vi "changeTempdatabase.vi"(3 "Database input(hidden)":T1={"DB name"="K2_r01", "UID"="mgupta", "password"="1qaz!QAZ"}) -> (0 "Database out":T1)   [LabVIEW 2016]
doc: "1/13/00, MG\nGrp: User\nFor intensity measurements\nAsks the user to input:\n1. Database name\n2. User Id\n3. Password"
uses:
  type def/Database.ctl
panel:
  in  "Boolean":bool
  in  "Database":T1={"DB name"="K2_r01", "UID"="sel02776", "password"="1qaz!QAZ"}
  in  "String":string
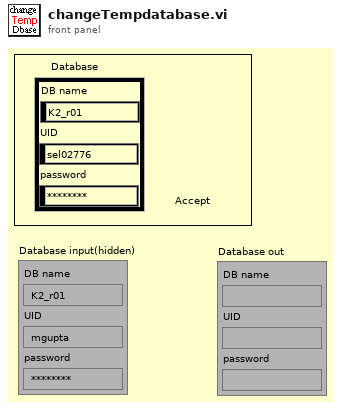
[diagram p1: front panel]
types:
  T1 = typedef "Database.ctl" = cluster{"DB name":string, "UID":string, "password":string}
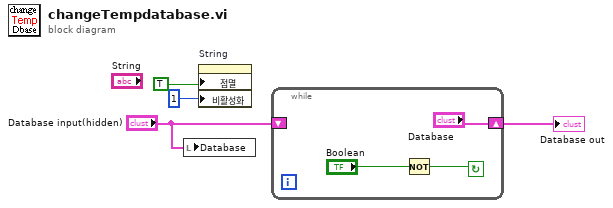
[diagram p0: block diagram]
diagram:
  n1 = local write "Database"("Database input(hidden)") -> ()
  n2 = property on="String" class="Str"("점멸"=TRUE ("Write Attribute"), "비활성화"=u8 1 ("Write Attribute")) -> ()  [unwired: 2 in, 2 out]
  n3 = while {
    shift-left: "Database input(hidden)" -> [_]
    shift-right: ["Database"] -> w3
    stop <- w7 continue-if-true
    n4 = Not(x="Boolean") -> (.not. x?=w7:bool)
  }
  "Database out" <- w3
